vi "TestView_Tree_Single_SoftFP.vi"(0 "reference in":refnum<class "TestView_Tree_Single.lvclass">, 2 "Floating":bool, 5 "error in (no error)":errorcluster) -> (14 "reference out":refnum<class "TestView_Tree_Single.lvclass">, 19 "error out":errorcluster)   [LabVIEW 2022 SP3, in "TestView_Tree_Single.lvlib" / "TestView_Tree_Single.lvclass"]
uses:
  TestView_Tree_Single.lvclass
  Components/ViPER.lvlibp/ViPER.lvclass
  C:/Projects/Medulla/ViPER/Examples/Flux_Capacitor_Tester/Components/ViPER.lvlibp/ViPER.lvclass
panel:
  out "Status":string
  out "Title":string
  out "Tree":string(tree)="1.0"
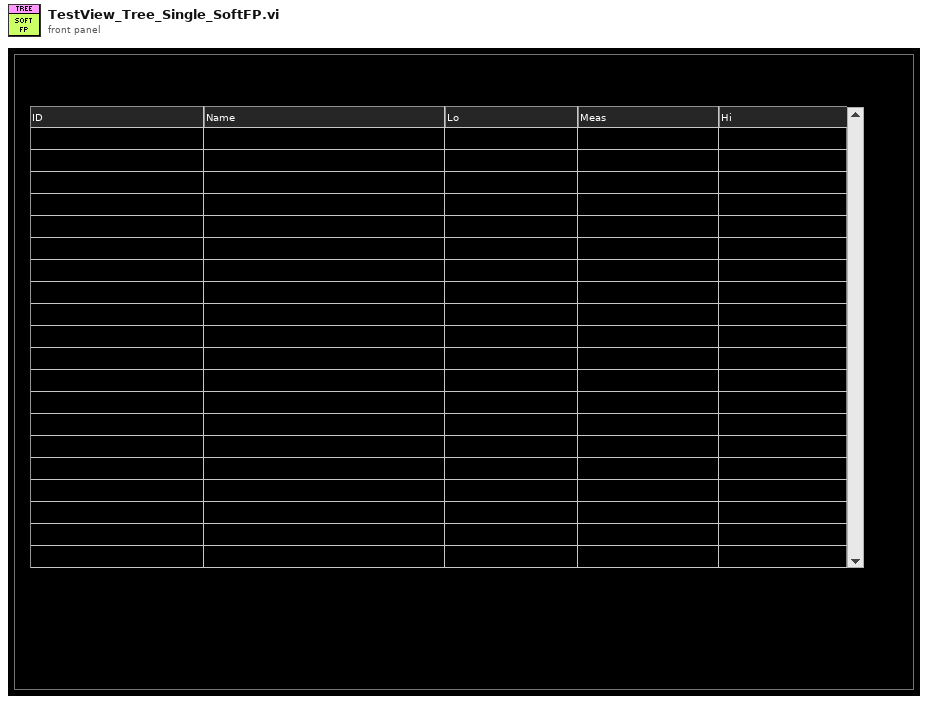
[diagram p1: front panel]
types:
  T1 = enum32{"Invalid", "Standard", "Closed", "Hidden", "Minimized", "Maximized"}
  T2 = typedef "TestView_Tree_Single.lvlib/TestView_Tree_Single.lvclass/ObjectAttributes.ctl" = cluster{"Front Panel":refnum<vi>, "Last_Item":string, "Config":T3, "Title":string, "User":string, "TreeRef":refnum<vi>, "Active DUT":i32, "Status":T4, "SN":string, "Spec":string}
  T3 = typedef "TestView_Tree_Single.lvlib/TestView_Tree_Single.lvclass/Config.ctl" = cluster{"default":string}
  T4 = typedef "TestView_Base.lvlibp/TestView_Base.lvclass/ViewStatus.ctl" = enum16{"Testing", "Ready", "Logout", "Login", "PASS", "FAIL", "FAULT", "ABORTED"}
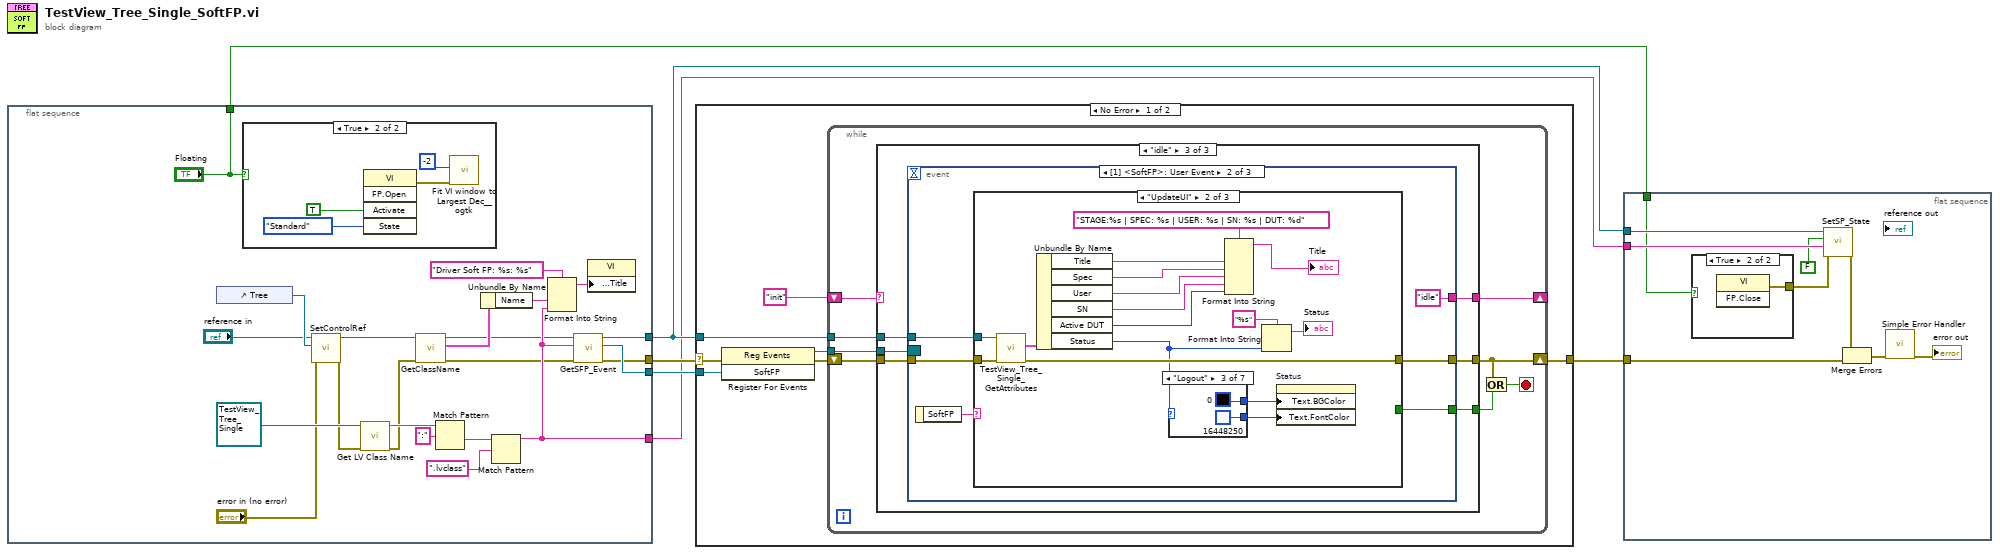
[diagram p0: block diagram]
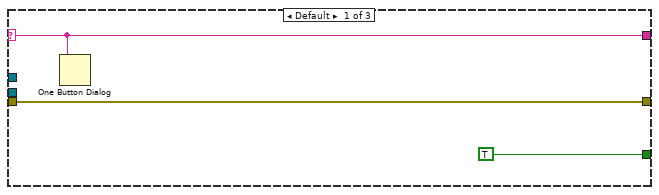
[diagram p4: hidden frame]
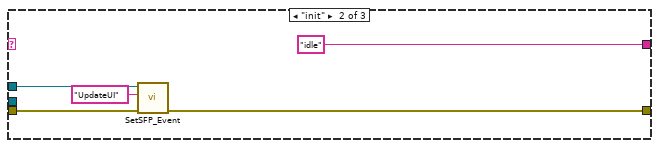
[diagram p5: hidden frame]
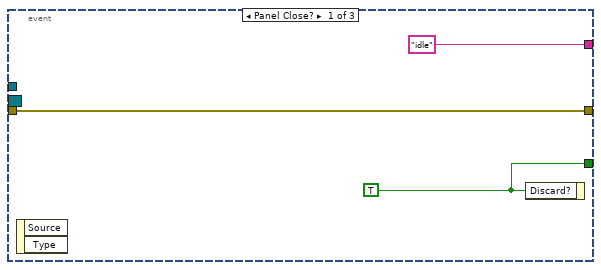
[diagram p6: hidden frame]
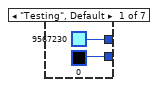
[diagram p8: hidden frame]
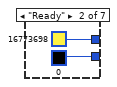
[diagram p9: hidden frame]
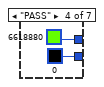
[diagram p10: hidden frame]
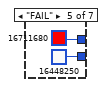
[diagram p11: hidden frame]
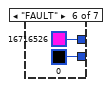
[diagram p12: hidden frame]
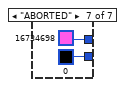
[diagram p13: hidden frame]
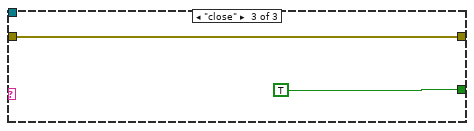
[diagram p14: hidden frame]
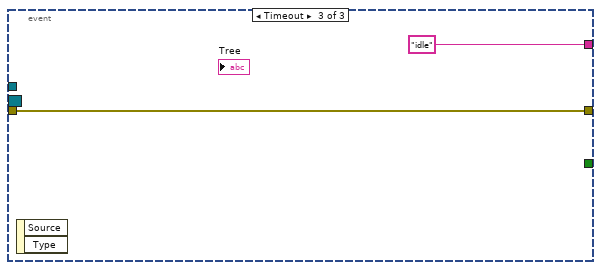
[diagram p15: hidden frame]
diagram:
  n1 = flat-sequence {
    tunnel: [w14] -> w6
    tunnel: [w13] -> w3
    tunnel: [w28] -> w4
    tunnel: [w20] -> w2
    tunnel: ["Floating"] -> w1
    frame #0 {
      n2 = control-ref of="Tree"() -> (w12:refnum<vi>)
      n3 = case shown="True" "Floating" {
        frame False {
        }
        frame True {
          n4 = invoke class="VI" method="FP.Open"("Activate"=TRUE ("Activate?"), "State"=T1."Standard") -> (error out=w29:errorcluster)  [unwired: 3 in, 4 out]
          n5 = call <userlib>:"Fit VI window to Largest Dec__ogtk.vi"("error in (no error)"=w29, "border spacing (2 px)"=-2) -> ()  [unwired: 4 in, 2 out]
        }
      }
      n6 = call-dynamic "SetControlRef.vi"("error in (no error)"="error in (no error)", "Ctl Ref"=w12, "reference in"="reference in") -> ("error out"=w8:errorcluster, "reference in"=w10:refnum<class "TestView_Tree_Single.lvclass">)  [unwired: 7 in]
      n7 = call <vilib>:"Get LV Class Name.vi"("error in (no error)"=w8, "object"=refnum<class "TestView_Tree_Single.lvclass"> refnum ("TestView_Tree.lvlib:TestView_Tree")) -> ("error out"=w19:errorcluster, "class name"=w23:string)  [unwired: 8 in]
      n8 = call "GetClassName.vi"("error in (no error)"=w19, "reference in"=w10) -> ("error out"=w18:errorcluster, "Details"=w17:cluster{"Name":string, "Class":string}, "reference out"=w16:refnum<class "TestView_Tree_Single.lvclass">)  [unwired: 7 in]
      n9 = Match Pattern(string=w23, regular expression=":") -> (after substring=w21:string)  [unwired: 1 in, 3 out]
      n10 = Unbundle By Name(w17) -> ("Name"=w25:string)
      n11 = Match Pattern(string=w21, regular expression=".lvclass") -> (before substring=w20:string)  [unwired: 1 in, 3 out]
      n12 = Format Into String(format string="Driver Soft FP: %s: %s", w25, w20) -> (resulting string=w27:string)  [unwired: 2 in, 1 out]
      n13 = call-dynamic "GetSFP_Event.vi"("error in (no error)"=w18, "Ancestor"=w20, "reference in"=w16) -> ("error out"=w14:errorcluster, "SoftFP"=w28:refnum<user-event>, "reference out"=w13:refnum<class "TestView_Tree_Single.lvclass">)  [unwired: 6 in]
      n14 = property class="VI"("Front Panel.Title"=w27) -> ()  [unwired: 2 in, 2 out]
    }
  }
  n15 = case shown="No Error" w6 {
    selector: w6 -> [w37 w106]
    tunnel: [w33 w106] -> w5
    tunnel: w3 -> [w34 _]
    tunnel: w4 -> [w39 _]
    frame No Error {
      n16 = register-events(error in=w37, w39) -> (reference out=w38:refnum<event-registration>, error out=w36:errorcluster)  [unwired: 1 in]
      n17 = while {
        shift-right: [w44] -> w33
        shift-left: w36 -> [w47]
        tunnel: w38 -> [w46]
        tunnel: w34 -> [w45]
        shift-right: [w40] -> _
        shift-left: "init" -> [w41]
        stop <- w43 stop-if-true
        n18 = case shown="\"idle\"" w41 {
          selector: w41 -> [w48 _ _]
          tunnel: w47 -> [w49 w54 w61]
          tunnel: w46 -> [_ _ w60]
          tunnel: w45 -> [_ w52 w59]
          tunnel: [w49 w53 w58] -> w44
          tunnel: [TRUE ("Discard?") _ w57] -> w42
          tunnel: [w48 "idle" w56] -> w40
          frame Default {
            n19 = One Button Dialog(message=w48) -> ()  [unwired: 1 in, 1 out]
          }
          frame "init" {
            n20 = call-dynamic "SetSFP_Event.vi"("error in (no error)"=w54, "msg"="UpdateUI", "reference in"=w52) -> ("error out"=w53:errorcluster)  [unwired: 7 in, 1 out]
          }
          frame "idle" {
            n21 = event shown="[1] <SoftFP>: User Event" {
              selector: w60 -> [_ _ _]
              dyn-events: _ -> [_ _ _]
              timeout: _ -> [_ _ _]
              tunnel: w61 -> [w64 w70 w105]
              tunnel: [w64 w68 w105] -> w58
              tunnel: [w63 w67 _] -> w57
              tunnel: w59 -> [_ w65 _]
              tunnel: ["idle" "idle" "idle"] -> w56
              event Panel Close? {
                w63 = TRUE ("Discard?")
                n22 = event-data() -> ()  [unwired: 1 in, 2 out]
                n23 = event-data("Discard?"=w63) -> ()  [unwired: 1 in, 1 out]
              }
              event User Event {
                n24 = event-data() -> ("SoftFP"=w69:string)  [unwired: 1 in]
                n25 = case shown="\"UpdateUI\"" w69 {
                  tunnel: w70 -> [w71 w87 w103]
                  tunnel: [w71 w85 w103] -> w68
                  tunnel: [_ _ TRUE ("Discard?")] -> w67
                  tunnel: w65 -> [_ w86 _]
                  frame Default {
                  }
                  frame "UpdateUI" {
                    n26 = call "TestView_Tree_Single_GetAttributes.vi"("error in (no error)"=w87, "reference in"=w86) -> ("error out"=w85:errorcluster, "Data"=w84:T2)  [unwired: 6 in, 2 out]
                    n27 = Unbundle By Name(w84) -> ("Title"=w76:string, "Spec"=w75:string, "User"=w74:string, "SN"=w73:string, "Active DUT"=w72:i32, "Status"=w79:T4)
                    n28 = case shown="\"Logout\"" w79 {
                      tunnel: [u32 9567230 ("Color Box") u32 16773698 ("Color Box") u32 0 ("Color Box") u32 6618880 ("Color Box") u32 16711680 ("Color Box") u32 16716526 ("Color Box") u32 16734698 ("Color Box")] -> w80
                      tunnel: [u32 0 ("Color Box") u32 0 ("Color Box") u32 16448250 ("Color Box") u32 0 ("Color Box") u32 16448250 ("Color Box") u32 0 ("Color Box") u32 0 ("Color Box")] -> w81
                      frame "Testing", Default {
                      }
                      frame "Ready" {
                      }
                      frame "Logout" {
                      }
                      frame "PASS" {
                      }
                      frame "FAIL" {
                      }
                      frame "FAULT" {
                      }
                      frame "ABORTED" {
                      }
                    }
                    n29 = Format Into String(format string="STAGE:%s | SPEC: %s | USER: %s | SN: %s | DUT: %d", w76, w75, w74, w73, w72) -> (resulting string=→"Title":string)  [unwired: 2 in, 1 out]
                    n30 = Format Into String(format string="%s", w79) -> (resulting string=→"Status":string)  [unwired: 2 in, 1 out]
                    n31 = property on="Status" class="Str"("Text.BGColor"=w80, "Text.FontColor"=w81) -> ()  [unwired: 2 in, 2 out]
                  }
                  frame "close" {
                  }
                }
              }
              event Timeout {
                n32 = event-data() -> ()  [unwired: 1 in, 2 out]
              }
            }
          }
        }
        n33 = Or(x=w44, y=w42) -> (x .or. y?=w43:bool)
      }
    }
    frame Error {
    }
  }
  n34 = flat-sequence {
    tunnel: w5 -> [w113]
    tunnel: w3 -> [w108]
    tunnel: w2 -> [w110]
    tunnel: w1 -> [w107]
    frame #0 {
      n35 = case shown="True" w107 {
        tunnel: [_ w116] -> w112
        frame False {
        }
        frame True {
          n36 = invoke class="VI" method="FP.Close"() -> (error out=w116:errorcluster)  [unwired: 3 in, 2 out]
        }
      }
      n37 = call "SetSP_State.vi"("error in (no error)"=w112, "Ancestor"=w110, "SP Open"=FALSE, "reference in"=w108) -> ("error out"=w111:errorcluster)  [unwired: 6 in, 1 out]
      n38 = Merge Errors(w111, w113) -> (w115:errorcluster)
      n39 = call <vilib>:"Simple Error Handler.vi"("error in (no error)"=w115) -> ("error out"=→"error out":errorcluster)  [unwired: 4 in, 4 out]
    }
  }
